vi "Write Multiple Channels with Simple Header.vi"() -> ()   [LabVIEW 2024]
doc: "The VI auto-generates a string based on date and time and opens a file using the date time string as a file name. An array containing a sine and square wave is converted to a tab delimited string and written to the file. The file is then closed."
uses:
  <vilib>/Analysis/NI_AALBase.lvlib
panel:
  in  "UUT Serial Number":string="A12345"
  in  "Operator Name":string="Leonardo DaVinci"
  out "Simulated Data":dbl[][](graph)
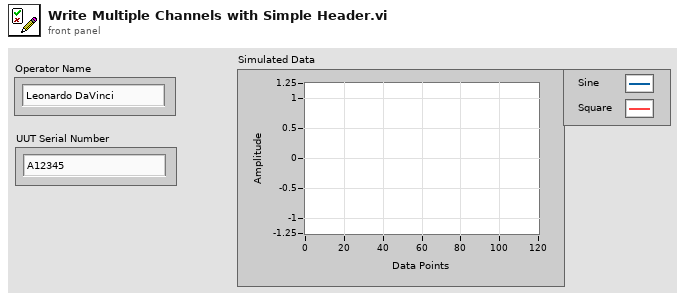
[diagram p1: front panel]
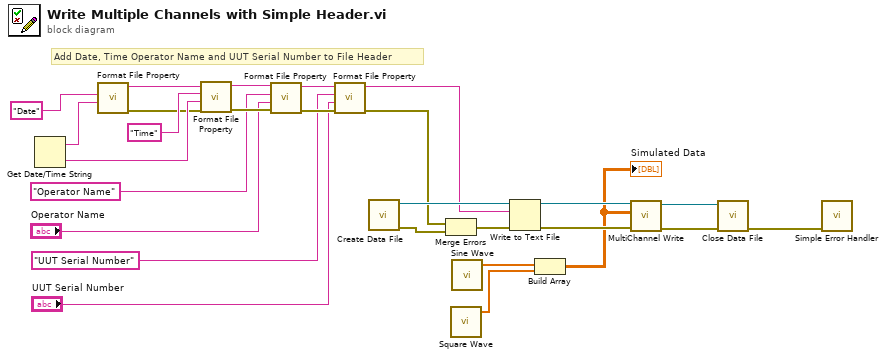
[diagram p0: block diagram]
diagram:
  # "Add Date, Time Operator Name and UUT Serial Number to File Header"
  n1 = Get Date/Time String() -> (date string=w24:string, time string=w21:string)  [unwired: 3 in]
  n2 = call "Format File Property.vi"("File Property Value"=w24, "File Property Name"="Date") -> ("Error Out"=w14:errorcluster, "String out"=w22:string)  [unwired: 8 in]
  n3 = call "Format File Property.vi"("Error In"=w14, "File Property Value"=w21, "File Property Name"="Time", "String in"=w22) -> ("Error Out"=w15:errorcluster, "String out"=w16:string)  [unwired: 6 in]
  n4 = call "Format File Property.vi"("Error In"=w15, "File Property Value"="Operator Name", "File Property Name"="Operator Name", "String in"=w16) -> ("Error Out"=w13:errorcluster, "String out"=w12:string)  [unwired: 6 in]
  n5 = call "Format File Property.vi"("Error In"=w13, "File Property Value"="UUT Serial Number", "File Property Name"="UUT Serial Number", "String in"=w12) -> ("Error Out"=w8:errorcluster, "String out"=w11:string)  [unwired: 6 in]
  n6 = call "Create Data File.vi"() -> ("Error Out"=w6:errorcluster, "File Refnum"=w20:refnum<file>)  [unwired: 10 in]
  n7 = Merge Errors(w8, w6) -> (w7:errorcluster)
  n8 = call <vilib>:"Square Wave.vi"() -> ("square wave"=w26:dbl[])  [unwired: 6 in, 2 out]
  n9 = call <vilib>:"Sine Wave.vi"() -> ("sine wave"=w27:dbl[])  [unwired: 5 in, 2 out]
  n10 = Write to Text File(file (use dialog)=w20, text=w11, error in=w7) -> (refnum out=w19:refnum<file>, error out=w18:errorcluster)  [unwired: 1 in, 1 out]
  n11 = Build Array(w27, w26) -> (w17:dbl[][])
  "Simulated Data" <- w17
  n12 = call "MultiChannel Write.vi"("Error In"=w18, "Data to Log"=w17, "File Refnum In"=w19) -> ("Error Out"=w3:errorcluster, "File Refnum Out"=w1:refnum<file>)  [unwired: 7 in]
  n13 = call "Close Data File.vi"("error in"=w3, "File Refnum In"=w1) -> ("error out"=w2:errorcluster)  [unwired: 9 in]
  n14 = call <vilib>:"Simple Error Handler.vi"("error in (no error)"=w2) -> ()  [unwired: 4 in, 5 out]
